vi "doCount.vi"(5 "counts_out_ref_chart":refnum<vi>, 7 "counts_out_ref":refnum<vi>, 8 "enable":refnum<vi>, 10 "Acquisition time [s]":dbl=0.1 format="%.3f", 11 "cursors_ref":refnum<vi>) -> ()   [LabVIEW 2014]
uses:
  <vilib>/Platform/TimedLoop/XDataNode/timing_clust.ctl
  <vilib>/Platform/TimedLoop/XDataNode/nitl_modes.ctl
  <vilib>/Platform/TimedLoop/XDataNode/wakeup.ctl
  dependencies/global_channels.vi
  <vilib>/platform/TimedLoop/XDataNode/XDataNode.xnode
  <vilib>/Platform/TimedLoop/XDataNode/XDNodeRunTimeDep.lvlib
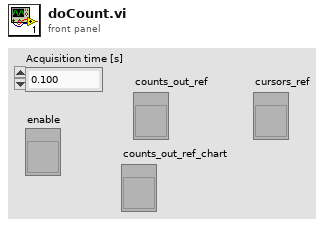
[diagram p1: front panel]
types:
  T1 = typedef "XDNodeRunTimeDep.lvlib/timing_clust.ctl" = cluster{"Expected End [f-1]":u64, "Actual End [f-1]":u64, "Finished Late? [f-1]":bool, "Expected End [i-1]":u64, "Actual End [i-1]":u64, "Finished Late? [i-1]":bool, "Expected Start [i]":u64, "Actual Start [i]":u64, "Expected Start [f]":u64, "Actual Start [f]":u64, "Source Name":string, "Structure Name":string, "Period":i64, "Deadline":i64, "Offset":i64, "Start":i64, "Priority":i32, "Timeout":i32, "Mode":T2, "Wakeup Reason":T3, "Error":errorcluster, "Source Type":string, "Secondary Source Type":string, "Global End Time":u64, "Global Start Time":u64, "Frame Duration":u64, "Iteration Duration":u64, "Assigned CPU":i32, "I/O Scan Engine Mode":u32}
  T2 = typedef "XDNodeRunTimeDep.lvlib/nitl_modes.ctl" = enum32{"No Change", "Process missed periods, maintain original phase", "Discard missed periods, maintain original phase", "Process missed periods, ignore original phase", "Discard missed periods, ignore original phase"}
  T3 = typedef "XDNodeRunTimeDep.lvlib/wakeup.ctl" = enum32{"Normal", "Aborted", "Asynchronous wakeup", "Timing source error", "Timed loop error", "Timeout"}
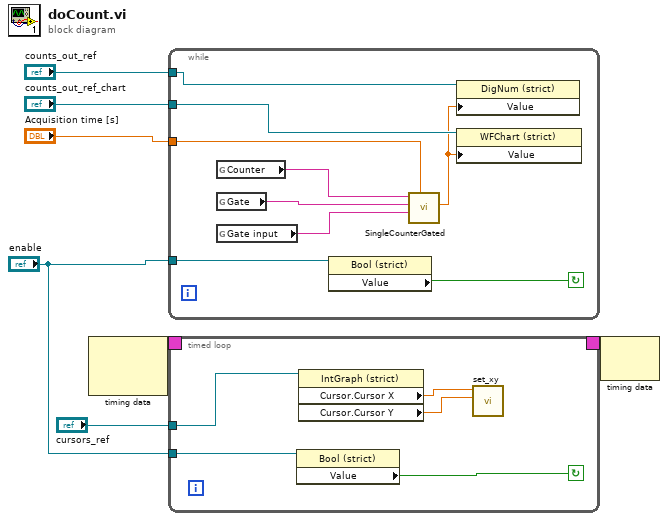
[diagram p0: block diagram]
diagram:
  n1 = node-c288() -> (w4:T1)  [unwired: 2 in]
  n2 = while {
    tunnel: "enable" -> [w13]
    tunnel: "counts_out_ref" -> [w12]
    tunnel: "Acquisition time [s]" -> [w11]
    tunnel: "counts_out_ref_chart" -> [w10]
    stop <- w8 continue-if-true
    n3 = global read "global_channels.vi" "Counter"() -> (w14:tag)
    n4 = global read "global_channels.vi" "Gate"() -> (w15:tag)
    n5 = global read "global_channels.vi" "Gate input"() -> (w16:tag)
    n6 = property class="Bool (strict)"(reference=w13) -> ("Value"=w8:bool)  [unwired: 1 in, 2 out]
    n7 = call "SingleCounterGated.vi"("Acquisition time [s]"=w11, "Gate input"=w16, "Gate"=w15, "Counter"=w14) -> ("counts/s"=w9:dbl)  [unwired: 5 in, 2 out]
    n8 = property class="DigNum (strict)"(reference=w12, "Value"=w9) -> ()  [unwired: 1 in, 2 out]
    n9 = property class="WFChart (strict)"(reference=w10, "Value"=w9) -> ()  [unwired: 1 in, 2 out]
  }
  n10 = timed-loop {
    timing: w4 -> [_]
    timing-out: [_] -> w3
    tunnel: "cursors_ref" -> [w19]
    tunnel: "enable" -> [w18]
    stop <- w17 continue-if-true
    n11 = property class="Bool (strict)"(reference=w18) -> ("Value"=w17:bool)  [unwired: 1 in, 2 out]
    n12 = property on="Property Node" class="IntGraph (strict)"(reference=w19) -> ("Cursor.Cursor X"=w21:dbl, "Cursor.Cursor Y"=w20:dbl)  [unwired: 1 in, 2 out]
    n13 = call "set_xy.vi"("y_value_um"=w20, "x_value_um"=w21) -> ()  [unwired: 9 in, 1 out]
  }
  n14 = node-c288(w3) -> ()  [unwired: 1 out]
